vi "autoDrive.vi"(1 "X Motion":dbl, 6 "Y Motion":dbl) -> (15 "finished?":bool, 23 "left speed":dbl, 24 "right speed":dbl, 25 "center speed":dbl)   [LabVIEW 2014]
doc: "Will drive the robot at a specified speed for a specified distance. Pretty simple."
uses:
  global variables/devrefs.vi
  <vilib>/addons/control/pid/pid.llb/PID (DBL).vi
  <vilib>/addons/control/pid/NI_PID_pid.lvlib
panel:
  out "Center Distance":dbl
  out "Left Distance":dbl
  out "Right Distance":dbl
  out "center desired rate":dbl format="%.2f"
  out "center rate":dbl
  out "right desired rate":dbl
  out "left desired rate":dbl
  out "left rate":dbl
  out "right rate":dbl
  # "Encoder Data"
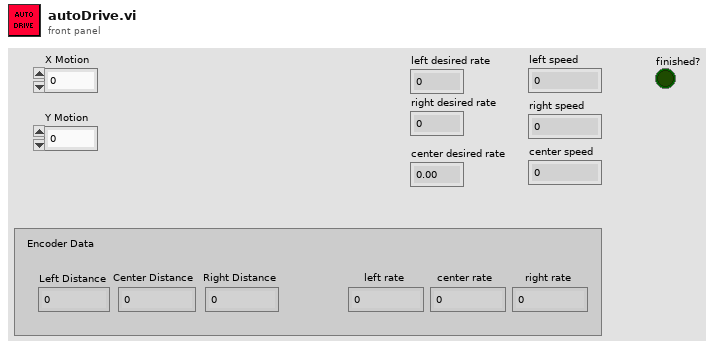
[diagram p1: front panel]
types:
  T1 = cluster{"proportional gain (Kc)":dbl, "integral time (Ti, min)":dbl, "derivative time (Td, min)":dbl}
  T2 = typedef "WPI_EncoderDevRef.ctl" = cluster{"DevStatus":errorcluster, "EncoderIndex":T3, "CounterIndex":T4, "DistancePerCount":dbl, "Decoding Type":T5}
  T3 = typedef "FPGA_EncoderIdx.ctl" = enum8{"Enc 0", "Enc 1", "Enc 2", "Enc 3", "Enc 4", "Enc 5", "Enc 6", "Enc 7", "Invalid"}
  T4 = typedef "FPGA_CounterCtrSystemIndex.ctl" = enum8{"Ctr 0", "Ctr 1", "Ctr 2", "Ctr 3", "Ctr 4", "Ctr 5", "Ctr 6", "Ctr 7", "Invalid"}
  T5 = typedef "WPI_EncoderType.ctl" = enum16{"1x", "2x", "4x"}
  T6 = typedef "subStates.ctl" = enum16{"null", "wait", "driver control", "auto", "manual override", "hold position", "rotate", "test", "end"}
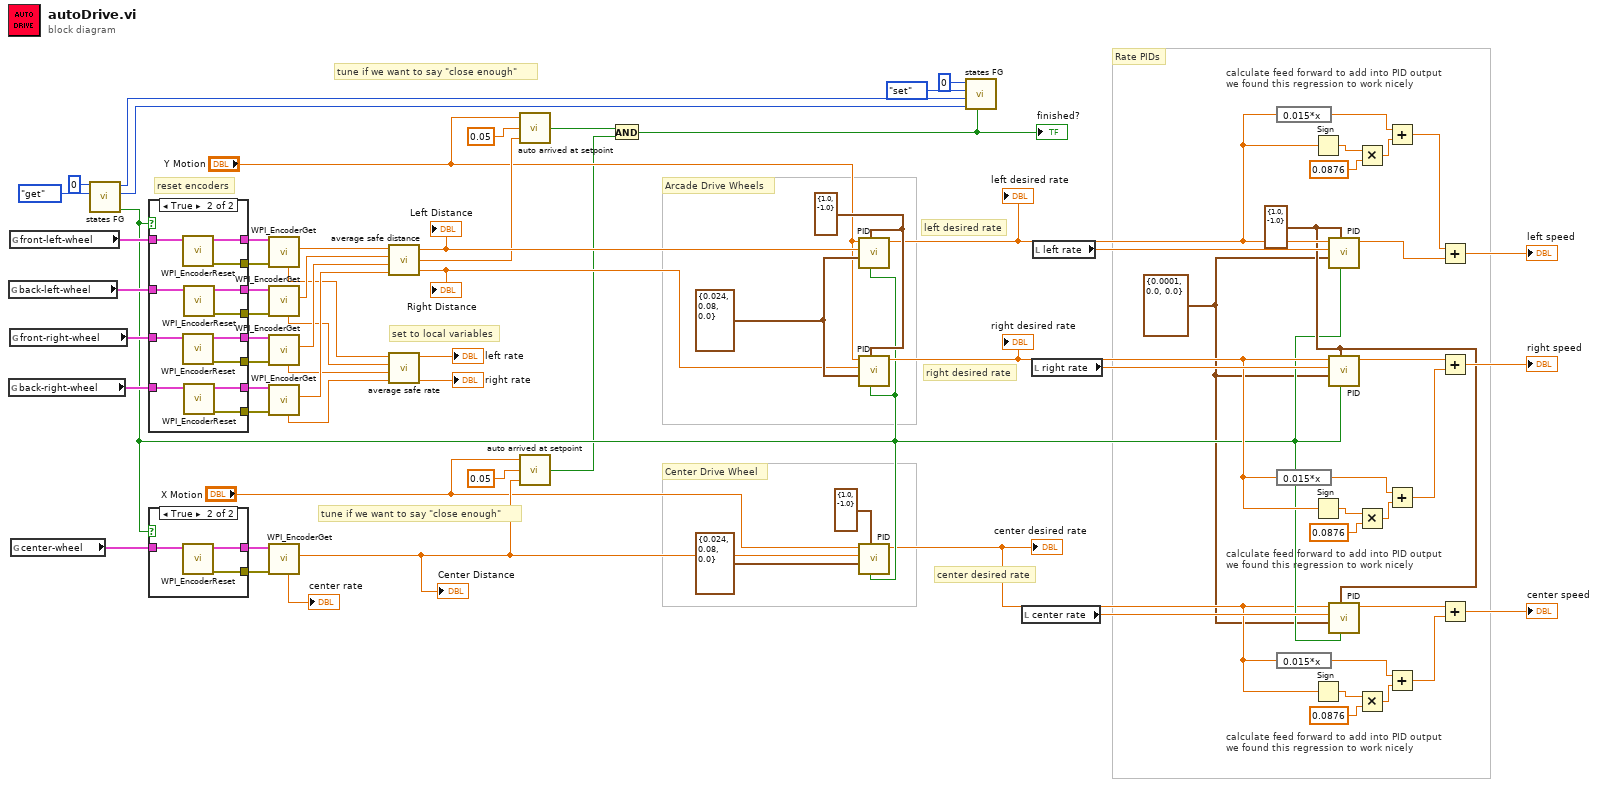
[diagram p0: block diagram]
diagram:
  w10 = T1 {"proportional gain (Kc)"=0.0001, "integral time (Ti, min)"=0.0, "derivative time (Td, min)"=0.0} ("Left Rate PID gains")
  w16 = cluster{"output high":dbl, "output low":dbl} {"output high"=1.0, "output low"=-1.0} ("output range")
  w31 = T1 {"proportional gain (Kc)"=0.024, "integral time (Ti, min)"=0.08, "derivative time (Td, min)"=0.0} ("Right Distance PID gains")
  w30 = cluster{"output high":dbl, "output low":dbl} {"output high"=1.0, "output low"=-1.0} ("output range")
  # "tune if we want to say \"close enough\""
  # "tune if we want to say \"close enough\""
  # "center desired rate"
  # "calculate feed forward to add into PID output\nwe found this regression to work nicely"
  # "set to local variables"
  # "Center Drive Wheel"
  # "reset encoders"
  # "Rate PIDs"
  # "calculate feed forward to add into PID output\nwe found this regression to work nicely"
  # "calculate feed forward to add into PID output\nwe found this regression to work nicely"
  # "Arcade Drive Wheels"
  # "left desired rate"
  # "right desired rate"
  n1 = global read "devrefs.vi" "back-left-wheel"() -> (w54:T2)
  n2 = global read "devrefs.vi" "back-right-wheel"() -> (w52:T2)
  n3 = global read "devrefs.vi" "front-left-wheel"() -> (w55:T2)
  n4 = global read "devrefs.vi" "front-right-wheel"() -> (w53:T2)
  n5 = global read "devrefs.vi" "center-wheel"() -> (w47:T2)
  n6 = call "states FG.vi"("menu (get)"=enum16{"set", "get"}."get", "Loop ID"=0) -> ("first call?"=w15:bool, "state # out"=w75:i32, "subState out"=w56:T6)  [unwired: 6 in, 1 out]
  n7 = case shown="True" w15 {
    tunnel: [_ w93] -> w50
    tunnel: [w78 w92] -> w51
    tunnel: [w79 w91] -> w49
    tunnel: [_ w90] -> w48
    tunnel: w55 -> [w78 w89]
    tunnel: w54 -> [w79 w88]
    tunnel: [_ w84] -> w46
    tunnel: [w80 w85] -> w45
    tunnel: [w81 w86] -> w43
    tunnel: [_ w87] -> w44
    tunnel: w53 -> [w80 w83]
    tunnel: w52 -> [w81 w82]
    frame False {
    }
    frame True {
      n8 = call <vilib>:"WPI_EncoderReset.vi"("EncoderDevRef"=w89) -> ("error out"=w93:errorcluster, "EncoderDevRef"=w92:T2)  [unwired: 9 in]
      n9 = call <vilib>:"WPI_EncoderReset.vi"("EncoderDevRef"=w83) -> ("error out"=w84:errorcluster, "EncoderDevRef"=w85:T2)  [unwired: 9 in]
      n10 = call <vilib>:"WPI_EncoderReset.vi"("EncoderDevRef"=w88) -> ("error out"=w90:errorcluster, "EncoderDevRef"=w91:T2)  [unwired: 9 in]
      n11 = call <vilib>:"WPI_EncoderReset.vi"("EncoderDevRef"=w82) -> ("error out"=w87:errorcluster, "EncoderDevRef"=w86:T2)  [unwired: 9 in]
    }
  }
  n12 = case shown="True" w15 {
    tunnel: [_ w97] -> w42
    tunnel: [w94 w96] -> w41
    tunnel: w47 -> [w94 w95]
    frame False {
    }
    frame True {
      n13 = call <vilib>:"WPI_EncoderReset.vi"("EncoderDevRef"=w95) -> ("error out"=w97:errorcluster, "EncoderDevRef"=w96:T2)  [unwired: 9 in]
    }
  }
  n14 = call <vilib>:"WPI_EncoderGet.vi"("error in (no error)"=w50, "EncoderDevRef"=w51) -> ("Distance"=w40:dbl, "Rate"=w33:dbl)  [unwired: 4 in, 4 out]
  n15 = call <vilib>:"WPI_EncoderGet.vi"("error in (no error)"=w48, "EncoderDevRef"=w49) -> ("Distance"=w39:dbl, "Rate"=w34:dbl)  [unwired: 4 in, 4 out]
  n16 = call <vilib>:"WPI_EncoderGet.vi"("error in (no error)"=w46, "EncoderDevRef"=w45) -> ("Distance"=w38:dbl, "Rate"=w35:dbl)  [unwired: 4 in, 4 out]
  n17 = call <vilib>:"WPI_EncoderGet.vi"("error in (no error)"=w44, "EncoderDevRef"=w43) -> ("Distance"=w37:dbl, "Rate"=w36:dbl)  [unwired: 4 in, 4 out]
  n18 = call <vilib>:"WPI_EncoderGet.vi"("error in (no error)"=w42, "EncoderDevRef"=w41) -> ("Distance"=w3:dbl, "Rate"=→"center rate":dbl)  [unwired: 4 in, 4 out]
  "Center Distance" <- w3
  n19 = call "average safe distance.vi"("Front Left"=w40, "Back Left"=w39, "Front Right"=w38, "Back Right"=w37) -> ("Left Distance"=w32:dbl, "Average Distance"=w7:dbl, "Right Distance"=w25:dbl)  [unwired: 2 in]
  "Right Distance" <- w25
  "Left Distance" <- w32
  n20 = call "average safe rate.vi"("Back Right"=w36, "Front Right"=w35, "Back Left"=w34, "Front Left"=w33) -> ("Right Average Rate"=→"right rate":dbl, "Left Average Rate"=→"left rate":dbl)  [unwired: 6 in]
  n21 = call "auto arrived at setpoint.vi"("Encoder Distance"=w7, "Tolerance"=0.05, "Setpoint"="Y Motion") -> ("At Location?"=w8:bool)
  n22 = call "auto arrived at setpoint.vi"("Encoder Distance"=w3, "Tolerance"=0.05, "Setpoint"="X Motion") -> ("At Location?"=w4:bool)
  n23 = And(x=w8, y=w4) -> (x .and. y?=w9:bool)
  "finished?" <- w9
  n24 = call-poly <vilib>:"PID.vi"("reinitialize? (F)"=w15, "output range"=w30, "PID gains"=w31, "process variable"=w32, "setpoint"="Y Motion") -> ("output"=w24:dbl)  [unwired: 5 in, 1 out]
  "left desired rate" <- w24
  n25 = call-poly <vilib>:"PID.vi"("reinitialize? (F)"=w15, "output range"=w30, "PID gains"=w31, "process variable"=w25, "setpoint"="Y Motion") -> ("output"=w23:dbl)  [unwired: 5 in, 1 out]
  "right desired rate" <- w23
  n26 = call-poly <vilib>:"PID.vi"("reinitialize? (F)"=w15, "output range"=cluster{"output high":dbl, "output low":dbl} {"output high"=1.0, "output low"=-1.0}, "PID gains"=T1 {"proportional gain (Kc)"=0.024, "integral time (Ti, min)"=0.08, "derivative time (Td, min)"=0.0} ("Right Distance PID gains"), "process variable"=w3, "setpoint"="X Motion") -> ("output"=w14:dbl)  [unwired: 5 in, 1 out]
  "center desired rate" <- w14
  n27 = call "states FG.vi"("exit in"=w9, "state # in"=w75, "subState in"=w56, "menu (get)"=enum16{"set", "get"}."set", "Loop ID"=0) -> ()  [unwired: 3 in, 4 out]
  n28 = local read "center rate"() -> (w17:dbl)
  n29 = local read "right rate"() -> (w71:dbl)
  n30 = local read "left rate"() -> (w72:dbl)
  n31 = expression code="0.015*x"(w24) -> (w63:dbl)
  n32 = expression code="0.015*x"(w23) -> (w60:dbl)
  n33 = expression code="0.015*x"(w14) -> (w18:dbl)
  n34 = Sign(1:w24) -> (0:w66:dbl)
  n35 = Sign(1:w23) -> (0:w57:dbl)
  n36 = Sign(1:w14) -> (0:w21:dbl)
  n37 = call-poly <vilib>:"PID.vi"("reinitialize? (F)"=w15, "output range"=w16, "PID gains"=w10, "process variable"=w72, "setpoint"=w24) -> ("output"=w62:dbl)  [unwired: 5 in, 1 out]
  n38 = call-poly <vilib>:"PID.vi"("reinitialize? (F)"=w15, "output range"=w16, "PID gains"=w10, "process variable"=w71, "setpoint"=w23) -> ("output"=w67:dbl)  [unwired: 5 in, 1 out]
  n39 = call-poly <vilib>:"PID.vi"("reinitialize? (F)"=w15, "output range"=w16, "PID gains"=w10, "process variable"=w17, "setpoint"=w14) -> ("output"=w13:dbl)  [unwired: 5 in, 1 out]
  n40 = Multiply(x=w66, y=0.0876) -> (x*y=w64:dbl)
  n41 = Multiply(x=w57, y=0.0876) -> (x*y=w59:dbl)
  n42 = Multiply(x=w21, y=0.0876) -> (x*y=w19:dbl)
  n43 = Add(x=w63, y=w64) -> (x+y=w61:dbl)
  n44 = Add(x=w60, y=w59) -> (x+y=w68:dbl)
  n45 = Add(x=w18, y=w19) -> (x+y=w12:dbl)
  n46 = Add(x=w61, y=w62) -> (x+y=→"left speed":dbl)
  n47 = Add(x=w67, y=w68) -> (x+y=→"right speed":dbl)
  n48 = Add(x=w13, y=w12) -> (x+y=→"center speed":dbl)
